vi "success_but_cant_real_time.vi"() -> ()   [LabVIEW 2018]
uses:
  <vilib>/imath/engines/lvmath2/RunTimeEngine/RangeToken/NIMS_Range.vi
  <instcachedir>/0/NIMS_Range_846134F467D14A349F7C6CCEF459CDB2.lvgen/NIMS_Range_846134F467D14A349F7C6CCEF459CDB2_000.vi
  <vilib>/imathl/engines/lvmath/Functions/Error Handling/Create Error.vi
  <vilib>/imath/engines/lvmath2/RunTimeEngine/BuiltInFunctions/length/NIMS_length(GV).vi
  <instcachedir>/0/NIMS_length(GV)_08A3D13377FD4E4B96F5795FBF3698FA.lvgen/NIMS_length(GV)_08A3D13377FD4E4B96F5795FBF3698FA_000.vi
  <vilib>/imath/engines/lvmath2/RunTimeEngine/BuiltInFunctions/inv/NIMS_inv(GM).vi
  <instcachedir>/0/NIMS_inv(GM)_A6DF8FE880224208AACFE4CF9F659502.lvgen/NIMS_inv(GM)_A6DF8FE880224208AACFE4CF9F659502_000.vi
  <vilib>/imath/engines/lvmath2/RunTimeEngine/ErrorHandling/NIMS_Error From Error Code.vi
  <vilib>/imath/engines/lvmath2/RunTimeEngine/BuiltInFunctions/zeros/NIMS_M=zeros(I32,I32).vi
  <vilib>/imath/engines/lvmath2/RunTimeEngine/RangeToken/NIMS_Range_R2 - Integer.vi
  <instcachedir>/0/NIMS_Range_R2 - Integer_E35B921DECF84AADB7325A02D418BFCC.lvgen/NIMS_Range_R2 - Integer_E35B921DECF84AADB7325A02D418BFCC_000.vi
  <vilib>/imath/engines/lvmath2/RunTimeEngine/CommandStatement/MC_CommandStatement_break.vi
  <vilib>/imath/engines/lvmath2/RunTimeEngine/IndexRead/NIMS M(S,S).vi
  <instcachedir>/0/NIMS M(S,S)_AC51E74150A542F7991B9634C66F3096.lvgen/NIMS M(S,S)_AC51E74150A542F7991B9634C66F3096_001.vi
  <vilib>/imath/engines/lvmath2/RunTimeEngine/BuiltInFunctions/abs/NIMS_abs(signed).vi
  <instcachedir>/0/NIMS_abs(signed)_C4FCB8E6058B49B797C7C8D53CA5F6EC.lvgen/NIMS_abs(signed)_C4FCB8E6058B49B797C7C8D53CA5F6EC_002.vi
  <vilib>/imath/engines/lvmath2/RunTimeEngine/BuiltInFunctions/atan2/NIMS_atan2.vi
  <instcachedir>/0/NIMS_atan2_A91AA4A7D42247EDBE8F76DB99AF04A4.lvgen/NIMS_atan2_A91AA4A7D42247EDBE8F76DB99AF04A4_001.vi
  <vilib>/imath/engines/lvmath2/RunTimeEngine/ErrorHandling/NIMS_Create Error From Enums.vi
  <vilib>/imath/engines/lvmath2/RunTimeEngine/BuiltInFunctions/asin/NIMS_asin(C).vi
  <instcachedir>/0/NIMS_asin(C)_AD59003138E84819B7347E9185C6620F.lvgen/NIMS_asin(C)_AD59003138E84819B7347E9185C6620F_001.vi
  <vilib>/imath/engines/lvmath2/RunTimeEngine/IndexRead/NIMS V(S).vi
  <instcachedir>/0/NIMS V(S)_0488751826AF41519A22953C041130DC.lvgen/NIMS V(S)_0488751826AF41519A22953C041130DC_003.vi
  <vilib>/imath/engines/lvmath2/RunTimeEngine/BuiltInFunctions/cos/NIMS_cos(C).vi
  <instcachedir>/0/NIMS_cos(C)_96B8A70E6B8E4D29AD8526A89C8CF3DF.lvgen/NIMS_cos(C)_96B8A70E6B8E4D29AD8526A89C8CF3DF_001.vi
  <vilib>/imath/engines/lvmath2/RunTimeEngine/BuiltInFunctions/sin/NIMS_sin(C).vi
  <instcachedir>/0/NIMS_sin(C)_7FE83C8DCD97403BBE687635FA1F837E.lvgen/NIMS_sin(C)_7FE83C8DCD97403BBE687635FA1F837E_001.vi
  <vilib>/imath/engines/lvmath2/RunTimeEngine/BuiltInFunctions/cross/NIMS_cross(GV,GV).vi
  <instcachedir>/0/NIMS_cross(GV,GV)_8E551EB9DC304C30866B49598818C259.lvgen/NIMS_cross(GV,GV)_8E551EB9DC304C30866B49598818C259_001.vi
  <vilib>/imath/engines/lvmath2/RunTimeEngine/ArithmeticOperatorToken/NIMS_ArithmeticOperator_multmx.vi
  <instcachedir>/0/NIMS_ArithmeticOperator_multmx_622CA76F9646436AB036D42A9A1CE0E6.lvgen/NIMS_ArithmeticOperator_multmx_622CA76F9646436AB036D42A9A1CE0E6_008.vi
  <vilib>/imath/engines/lvmath2/RunTimeEngine/BuiltInFunctions/cross/NIMS_cross(GM,GM,I32).vi
  <instcachedir>/0/NIMS_cross(GM,GM,I32)_0F6D45CF7D834A0BB6695B819A7F63BC.lvgen/NIMS_cross(GM,GM,I32)_0F6D45CF7D834A0BB6695B819A7F63BC_001.vi
  <vilib>/imath/engines/lvmath2/RunTimeEngine/ArithmeticOperatorToken/NIMS_ArithmeticOperator_plus.vi
  <instcachedir>/0/NIMS_ArithmeticOperator_plus_DE670E32103C4C10ADF2A97367172B30.lvgen/NIMS_ArithmeticOperator_plus_DE670E32103C4C10ADF2A97367172B30_002.vi
  <vilib>/imath/engines/lvmath2/RunTimeEngine/IndexRead/NIMS M(S).vi
  <instcachedir>/0/NIMS M(S)_B826C018497E4940AE96BD27B540B6FB.lvgen/NIMS M(S)_B826C018497E4940AE96BD27B540B6FB_004.vi
  <vilib>/imath/engines/lvmath2/RunTimeEngine/ArithmeticOperatorToken/NIMS_ArithmeticOperator_multmx(M,CV)-internal.vi
  <instcachedir>/0/NIMS_ArithmeticOperator_multmx(M,CV)-internal_5287250D8D1D4A3E9F77F5DF08D432E0.lvgen/NIMS_ArithmeticOperator_multmx(M,CV)-internal_5287250D8D1D4A3E9F77F5DF08D432E0_002.vi
  <vilib>/imath/engines/lvmath2/RunTimeEngine/BuiltInFunctions/norm/NIMS_norm(GV,DBL).vi
  <instcachedir>/0/NIMS_norm(GV,DBL)_D46CFC66D3594E6EB2AF828D88BCFE7F.lvgen/NIMS_norm(GV,DBL)_D46CFC66D3594E6EB2AF828D88BCFE7F_001.vi
  <vilib>/imath/engines/lvmath2/RunTimeEngine/ArithmeticOperatorToken/NIMS_ArithmeticOperator_power(S).vi
  <instcachedir>/0/NIMS_ArithmeticOperator_power(S)_E7916602C36D4BDA819D832F61F93EE1.lvgen/NIMS_ArithmeticOperator_power(S)_E7916602C36D4BDA819D832F61F93EE1_010.vi
  <vilib>/imath/engines/lvmath2/RunTimeEngine/IndexReplace/NIMS M(S,S)=S.vi
  <instcachedir>/0/NIMS M(S,S)=S_5DAF17B45D8A4C8588C7CF468644990A.lvgen/NIMS M(S,S)=S_5DAF17B45D8A4C8588C7CF468644990A_001.vi
  <vilib>/imath/engines/lvmath2/RunTimeEngine/IndexReplace/NIMS M($,S)=M.vi
  <instcachedir>/0/NIMS M($,S)=M_8628C75F074A456F99DEE5F6C7D1B8A6.lvgen/NIMS M($,S)=M_8628C75F074A456F99DEE5F6C7D1B8A6_001.vi
  <vilib>/imath/engines/lvmath2/RunTimeEngine/IndexReplace/NIMS M($,S)=V.vi
  <instcachedir>/0/NIMS M($,S)=V_C45C2B1F89AE4A41BE90F9497F10C990.lvgen/NIMS M($,S)=V_C45C2B1F89AE4A41BE90F9497F10C990_000.vi
  <vilib>/imath/engines/lvmath2/RunTimeEngine/VariableToken/NIMS_VariableToken_CondDefined.vi
  <instcachedir>/0/NIMS_VariableToken_CondDefined_BADDB804EBCA4B86883699DABD34B224.lvgen/NIMS_VariableToken_CondDefined_BADDB804EBCA4B86883699DABD34B224_000.vi
  <vilib>/imath/engines/lvmath2/RunTimeEngine/NodeEndStatement/NIMS_NodeEndStatement_Get Vector.vi
  <instcachedir>/0/NIMS_NodeEndStatement_Get Vector_329D0992E87F49F089135171B7FC9327.lvgen/NIMS_NodeEndStatement_Get Vector_329D0992E87F49F089135171B7FC9327_003.vi
  <vilib>/imath/engines/lvmath/Functions/Error Handling/MergeErrorsWrapper.vi
  <vilib>/imath/engines/lvmath2/RunTimeEngine/NodeEndStatement/NIMS_NodeEndStatement_Output.vi
  <instcachedir>/0/NIMS_NodeEndStatement_Output_53EC0D466D134D7ABD903AC30B43404B.lvgen/NIMS_NodeEndStatement_Output_53EC0D466D134D7ABD903AC30B43404B_005.vi
  <instcachedir>/0/NIMS_NodeEndStatement_Output_53EC0D466D134D7ABD903AC30B43404B.lvgen/NIMS_NodeEndStatement_Output_53EC0D466D134D7ABD903AC30B43404B_000.vi
  <vilib>/imath/engines/lvmath2/RunTimeEngine/ErrorHandling/NIMS_Finalize Error.vi
panel:
  out "W":dbl[](array[numeric])
  out "E":cdb[](array[numeric])
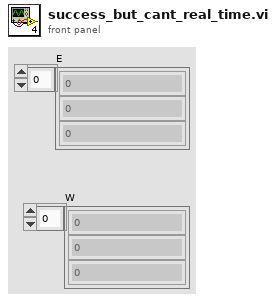
[diagram p1: front panel]
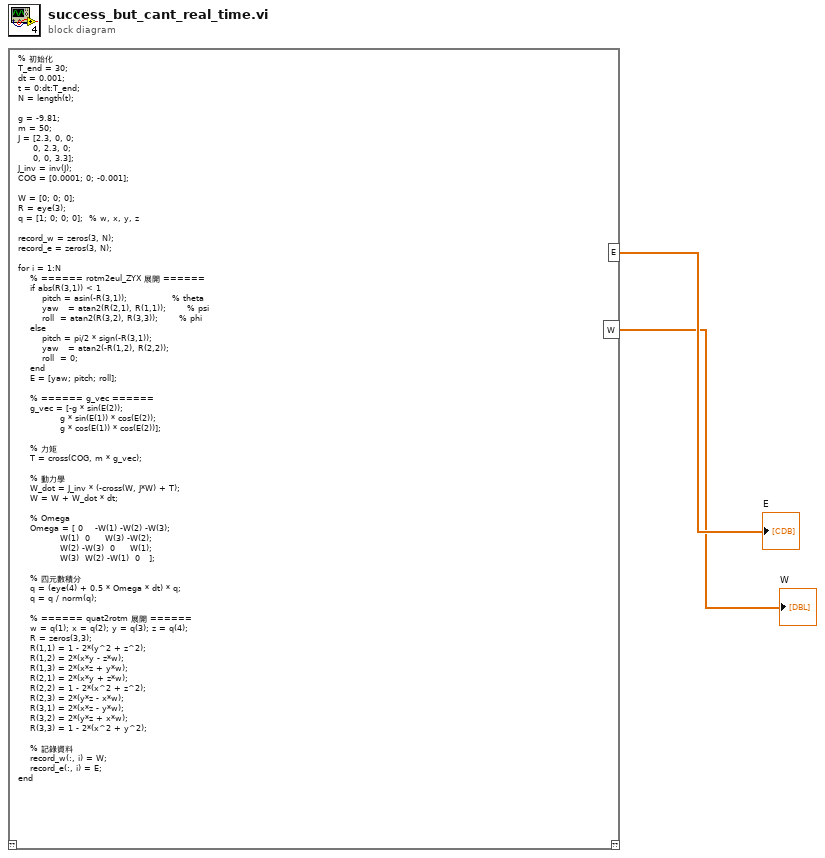
[diagram p0: block diagram]
diagram:
  n1 = mathscript code="% 初始化\nT_end = 30;\ndt = 0.001;\nt = 0:dt:T_end;\nN = length(t);\n\ng = -9.81;\nm = 50;\nJ = [2.3, 0, 0;\n     0, 2.3, 0;\n     0, 0, 3.3];\nJ_inv = inv(J);\nCOG = [0.0001; 0; -0.001];\n\nW = [0; 0; 0];\nR = eye(3);\nq = [1; 0; 0; 0];  % w, x, y, z\n\nrecord_w = zeros(3, N);\nrecord_e = zeros(3, N);\n\nfor i = 1:N\n    % ====== rotm2eul_ZYX 展開 ======\n    if abs(R(3,1)) < 1\n        pitch = asin(-R(3,1));               % theta\n        yaw   = atan2(R(2,1), R(1,1));       % psi\n        roll  = atan2(R(3,2), R(3,3));       % phi\n    else\n        pitch = pi/2 * sign(-R(3,1));\n        yaw   = atan2(-R(1,2), R(2,2));\n        roll  = 0;\n    end\n    E = [yaw; pitch; roll];\n\n    % ====== g_vec ======\n    g_vec = [-g * sin(E(2));\n              g * sin(E(1)) * cos(E(2));\n              g * cos(E(1)) * cos(E(2))];\n\n    % 力矩\n    T = cross(COG, m * g_vec);\n\n    % 動力學\n    W_dot = J_inv * (-cross(W, J*W) + T);\n    W = W + W_dot * dt;\n\n    % Omega\n    Omega = [ 0    -W(1) -W(2) -W(3);\n              W(1)  0     W(3) -W(2);\n              W(2) -W(3)  0     W(1);\n              W(3)  W(2) -W(1)  0   ];\n\n    % 四元數積分\n    q = (eye(4) + 0.5 * Omega * dt) * q;\n    q = q / norm(q);\n\n    % ====== quat2rotm 展開 ======\n    w = q(1); x = q(2); y = q(3); z = q(4);\n    R = zeros(3,3);\n    R(1,1) = 1 - 2*(y^2 + z^2);\n    R(1,2) = 2*(x*y - z*w);\n    R(1,3) = 2*(x*z + y*w);\n    R(2,1) = 2*(x*y + z*w);\n    R(2,2) = 1 - 2*(x^2 + z^2);\n    R(2,3) = 2*(y*z - x*w);\n    R(3,1) = 2*(x*z - y*w);\n    R(3,2) = 2*(y*z + x*w);\n    R(3,3) = 1 - 2*(x^2 + y^2);\n\n    % 記錄資料\n    record_w(:, i) = W;\n    record_e(:, i) = E;\nend"() -> ("E"=→"E":cdb[], "W"=→"W":dbl[])  [unwired: 1 in, 1 out]
